vi "Run.vi"(8 "error in (no error)":errorcluster, 9 "Interlock Chain":refnum<class "Interlock Chain.lvclass">, 11 "Cylinder in":refnum<class "Cylinder.lvclass">) -> (0 "error out":errorcluster, 3 "Cylinder out":refnum<class "Cylinder.lvclass">)   [LabVIEW 2015, in "cRIO-Carbondioxide.lvlib" / "CO2-Actor.lvlib" / "Cylinder.lvclass"]
uses:
  Cylinder.lvclass
  Interlocks/Interlock Chain/Interlock Chain.lvclass
  <vilib>/ActorFramework/Actor/Actor.lvclass/Actor.ctl
  <vilib>/ActorFramework/Message Enqueuer/Message Enqueuer.lvclass/Message Enqueuer.ctl
  Cylinder.lvclass/Cylinder.ctl
  <vilib>/ActorFramework/Actor/Read Self Enqueuer.vi
  <vilib>/ActorFramework/Message Enqueuer/Init from Existing Queue.vi
  <vilib>/ActorFramework/Actor/Actor.lvclass
  <vilib>/ActorFramework/Message Enqueuer/Message Enqueuer.lvclass
  CO2 Actor/CO2 Actor.lvclass
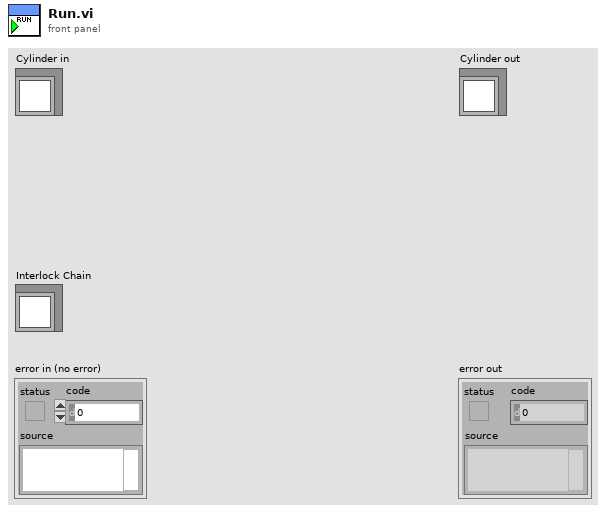
[diagram p1: front panel]
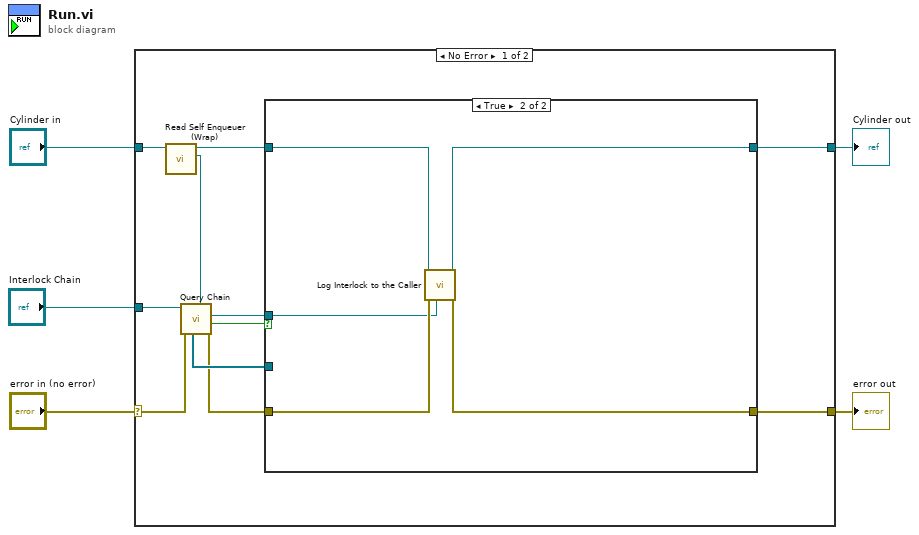
[diagram p0: block diagram]
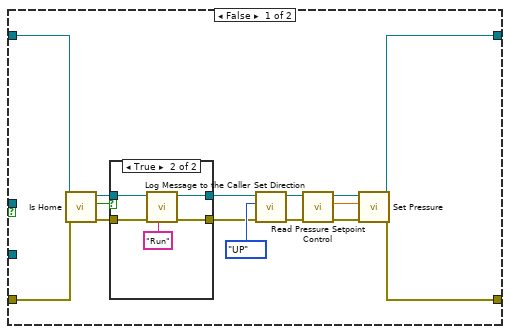
[diagram p2: hidden frame]
diagram:
  n1 = case shown="No Error" "error in (no error)" {
    selector: "error in (no error)" -> [w15 w45]
    tunnel: [w13 w45] -> w4
    tunnel: [w14 w44] -> w2
    tunnel: "Cylinder in" -> [w8 w44]
    tunnel: "Interlock Chain" -> [w16 _]
    frame No Error {
      n2 = call "Read Self Enqueuer (Wrap).vi"("CO2 Actor in"=w8) -> ("Actor Framework:Message Enqueuer"=w6:refnum<class "Message Enqueuer.lvclass">, "CO2 Actor out"=w7:refnum<class "Cylinder.lvclass">)  [unwired: 9 in]
      n3 = call "Query Chain.vi"("Caller Enqueuer"=w6, "error in (no error)"=w15, "Interlock Chain"=w16) -> ("error out"=w9:errorcluster, "Interlock?"=w10:bool, "Interlock out"=w12:refnum<class "Interlock.lvclass">, "IL Action"=w11:refnum<class "IL Action.lvclass">[])  [unwired: 3 in, 2 out]
      n4 = case shown="True" w10 {
        tunnel: w7 -> [w26 w43]
        tunnel: [w18 w40] -> w14
        tunnel: w9 -> [w28 w42]
        tunnel: [w17 w39] -> w13
        tunnel: w12 -> [_ w41]
        tunnel: w11 -> [_ _]
        frame False {
          n5 = call "Is Home.vi"("error in (no error)"=w28, "Cylinder in"=w26) -> ("error out"=w27:errorcluster, "Cylinder is Home"=w24:bool, "Cylinder out"=w25:refnum<class "Cylinder.lvclass">)  [unwired: 6 in, 1 out]
          n6 = case shown="True" w24 {
            tunnel: [w32 w38] -> w20
            tunnel: [w33 w37] -> w21
            tunnel: w27 -> [w32 w35]
            tunnel: w25 -> [w33 w34]
            frame False {
            }
            frame True {
              n7 = call-dynamic "Log Message to the Caller.vi"("String (\"\" = no message to send)"="Run" ("String (\"\" = no message to send)"), "error in (no error)"=w35, "CO2 Actor in"=w34) -> ("error out"=w38:errorcluster, "CO2 Actor out"=w37:refnum<class "Cylinder.lvclass">)  [unwired: 7 in]
            }
          }
          n8 = call "Set Direction.vi"("error in (no error)"=w20, "Direction (Down)"=enum16{"UP", "DOWN"}."UP", "Cylinder in"=w21) -> ("error out"=w19:errorcluster, "Cylinder out"=w22:refnum<class "Cylinder.lvclass">)  [unwired: 7 in]
          n9 = call "Read Pressure Setpoint Control .vi"("error in (no error)"=w19, "Cylinder in"=w22) -> ("error out"=w31:errorcluster, "Pressure Setpoint"=w29:dbl, "Cylinder out"=w30:refnum<class "Cylinder.lvclass">)  [unwired: 7 in]
          n10 = call "Set Pressure.vi"("error in (no error)"=w31, "Pressure (bar)"=w29, "Cylinder in"=w30) -> ("error out"=w17:errorcluster, "Cylinder out"=w18:refnum<class "Cylinder.lvclass">)  [unwired: 7 in]
        }
        frame True {
          n11 = call-dynamic "Log Interlock to the Caller.vi"("Interlock in"=w41, "error in (no error)"=w42, "CO2 Actor in"=w43) -> ("error out"=w39:errorcluster, "CO2 Actor out"=w40:refnum<class "Cylinder.lvclass">)  [unwired: 7 in]
        }
      }
    }
    frame Error {
    }
  }
  "error out" <- w4
  "Cylinder out" <- w2
